vi "Example CaseStructure 3.vi"(8 "Error In start":errorcluster) -> (0 "Error Out stop":errorcluster, 1 "signal out":waveform(dbl), 3 "appended array":waveform(dbl)[](array[waveform]))   [LabVIEW 2014]
uses:
  <vilib>/measure/NI_MABase.lvlib
panel:
  out "String":string
  in  "case string":string
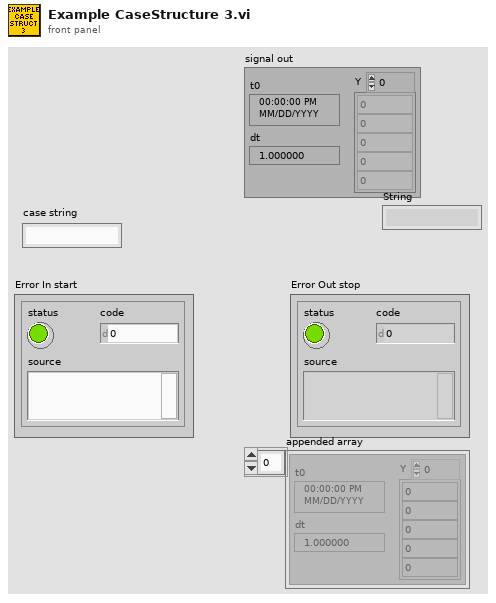
[diagram p1: front panel]
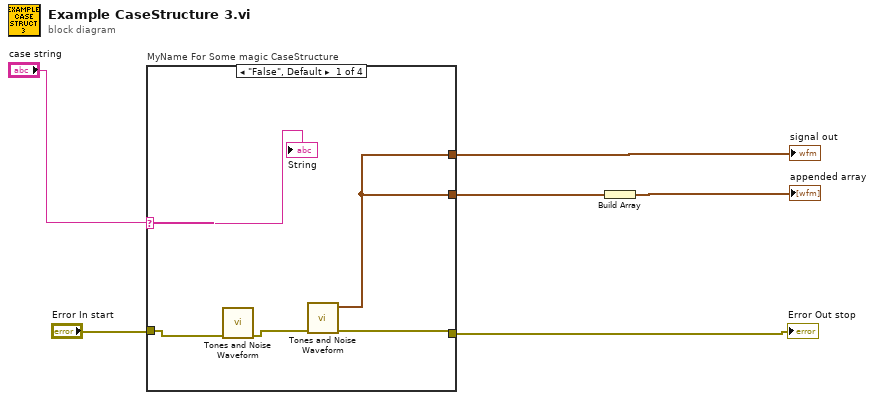
[diagram p0: block diagram]
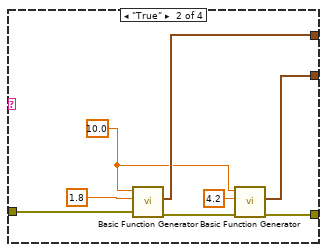
[diagram p2: hidden frame]
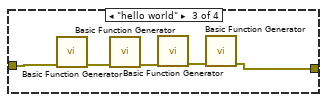
[diagram p3: hidden frame]
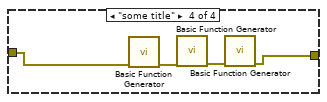
[diagram p4: hidden frame]
diagram:
  n1 = case "MyName For Some magic CaseStructure" shown="\"False\", Default" "case string" {
    selector: "case string" -> [w9 _ _ _]
    tunnel: "Error In start" -> [w8 w19 w24 w26]
    tunnel: [w11 w17 w20 w25] -> w2
    tunnel: [w10 w14 _ _] -> w5
    tunnel: [w10 w13 _ _] -> w4
    frame "False", Default {
      n2 = call <vilib>:"Tones and Noise Waveform.vi"("error in (no error)"=w8) -> ("error out"=w7:errorcluster)  [unwired: 9 in, 1 out]
      n3 = call <vilib>:"Tones and Noise Waveform.vi"("error in (no error)"=w7) -> ("error out"=w11:errorcluster, "signal out"=w10:waveform(dbl))  [unwired: 9 in]
      "String" <- w9
    }
    frame "True" {
      w12 = 10.0 ("frequency")
      n4 = call <vilib>:"Basic Function Generator.vi"("error in (no error)"=w19, "amplitude"=1.8, "frequency"=w12) -> ("error out"=w18:errorcluster, "signal out"=w14:waveform(dbl))  [unwired: 6 in, 1 out]
      n5 = call <vilib>:"Basic Function Generator.vi"("error in (no error)"=w18, "amplitude"=4.2, "frequency"=w12) -> ("error out"=w17:errorcluster, "signal out"=w13:waveform(dbl))  [unwired: 6 in, 1 out]
    }
    frame "hello world" {
      n6 = call <vilib>:"Basic Function Generator.vi"("error in (no error)"=w24) -> ("error out"=w21:errorcluster)  [unwired: 8 in, 2 out]
      n7 = call <vilib>:"Basic Function Generator.vi"("error in (no error)"=w21) -> ("error out"=w23:errorcluster)  [unwired: 8 in, 2 out]
      n8 = call <vilib>:"Basic Function Generator.vi"("error in (no error)"=w23) -> ("error out"=w22:errorcluster)  [unwired: 8 in, 2 out]
      n9 = call <vilib>:"Basic Function Generator.vi"("error in (no error)"=w22) -> ("error out"=w20:errorcluster)  [unwired: 8 in, 2 out]
    }
    frame "some title" {
      n10 = call <vilib>:"Basic Function Generator.vi"("error in (no error)"=w26) -> ("error out"=w28:errorcluster)  [unwired: 8 in, 2 out]
      n11 = call <vilib>:"Basic Function Generator.vi"("error in (no error)"=w28) -> ("error out"=w27:errorcluster)  [unwired: 8 in, 2 out]
      n12 = call <vilib>:"Basic Function Generator.vi"("error in (no error)"=w27) -> ("error out"=w25:errorcluster)  [unwired: 8 in, 2 out]
    }
  }
  "Error Out stop" <- w2
  "signal out" <- w5
  n13 = Build Array(w4) -> (→"appended array":waveform(dbl)[])
